vi "BRig_dataMTrig_Audio_T_L.vi"() -> (2 "output_Audio_T_L":i32)   [LabVIEW 2014]
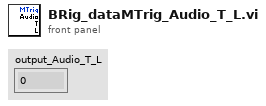
[diagram p1: front panel]
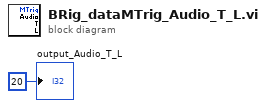
[diagram p0: block diagram]
diagram:
  "output_Audio_T_L" <- 20 ("output_iBlock")
